vi "Initialize Kinect.vi"(8 "error in (no error)":errorcluster, 9 "Depth Image Format":T1, 10 "Color Image Format":T2, 11 "Kinect Sensor Index":i32) -> (0 "error out":errorcluster, 3 "Kinect Session out":refnum<class "Kinect Session.lvclass">)   [LabVIEW 2014, in "Kinect Library.lvlib"]
doc: "This is the basic initialization VI for the Kinect API. You may use it to connect to any Kinect sensors attached to this computer. You can provide it with the index of the Kinect which can be retrieved using the Get Device Info VI."
uses:
  Kinect Library.lvlib
  Kinect Session Class/Kinect Session.lvclass
  Kinect Type Defs/Color Image Format.ctl
  Kinect Type Defs/Depth Image Format.ctl
  Microsoft.Kinect
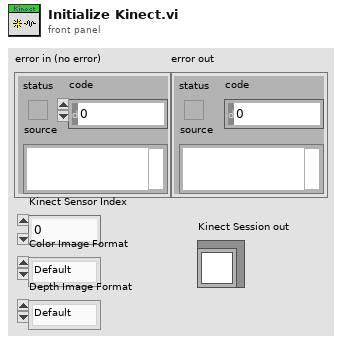
[diagram p1: front panel]
types:
  T1 = typedef "Kinect Library.lvlib/Depth Image Format.ctl" = enum16{"Default", "Undefined", "Resolution640x480Fps30", "Resolution320x240Fps30", "Resolution80x60Fps30"}
  T2 = typedef "Kinect Library.lvlib/Color Image Format.ctl" = enum16{"Default", "Undefined", "RgbResolution640x480Fps30", "RgbResolution1280x960Fps12", "YuvResolution640x480Fps15", "RawYuvResolution640x480Fps15"}
  T3 = cluster{"FramePixelDataLength":i32, "FrameWidth":i32, "FrameHeight":i32}
  T4 = cluster{"Skeleton Array":refnum<k24>[], "FrameSkeletonArrayLength":i32}
  T5 = typedef "Image Type" = u32
  T6 = typedef "IMAQ Image.ctl" = refnum<image>
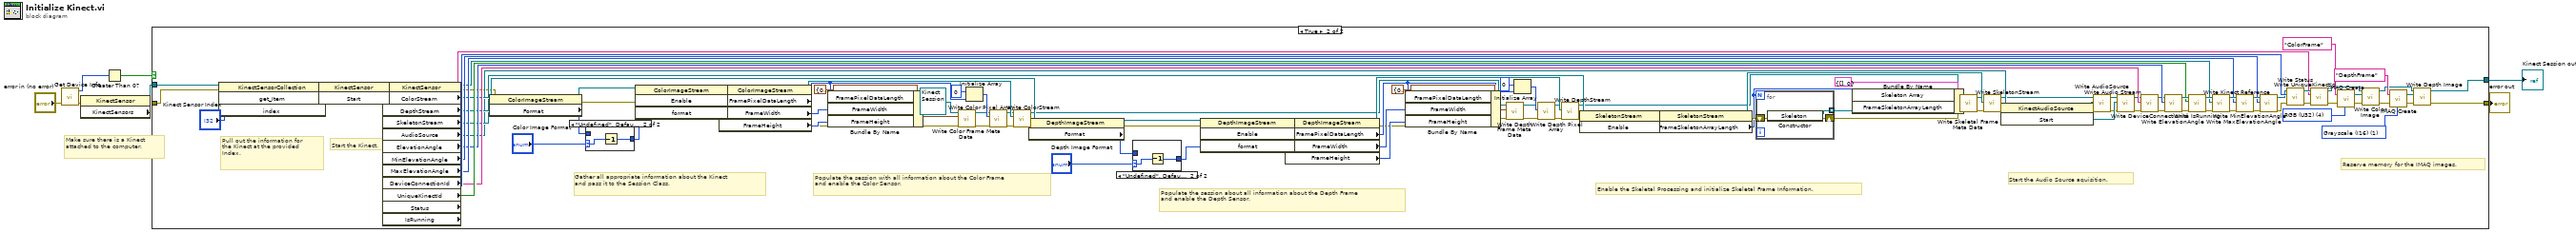
[diagram p0: block diagram]
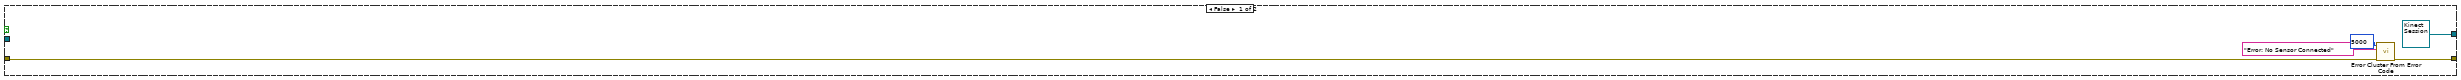
[diagram p2: hidden frame]
diagram:
  # "Make sure there is a Kinect\nattached to the computer."
  n1 = call "Get Device Info.vi"("error in (no error)"="error in (no error)") -> ("error out"=w4:errorcluster, "Number of Kinects Attached"=w8:i32)  [unwired: 8 in, 1 out]
  n2 = property class="KinectSensor"(error in=w4) -> (error out=w3:errorcluster, "KinectSensors"=w5:refnum<k24>)  [unwired: 1 in, 1 out]
  n3 = Greater Than 0?(x=w8) -> (x > 0?=w7:bool)
  n4 = case shown="True" w7 {
    tunnel: w3 -> [w11 w124]
    tunnel: w5 -> [_ w123]
    tunnel: [w10 w49] -> w1
    tunnel: [refnum<class "Kinect Session.lvclass"> refnum ("Kinect Session.lvclass") w46] -> w2
    frame False {
      n5 = call <vilib>:"Error Cluster From Error Code.vi"("error in (no error)"=w11, "error message (\"\")"="Error: No Sensor Connected" ("error message (\"\")"), "error code (0)"=5000) -> ("error out"=w10:errorcluster)  [unwired: 6 in]
    }
    frame True {
      w54 = T5 1 items=["Grayscale (U8)", "Grayscale (I16)", "Grayscale (SGL)", "Complex (CSG)", "RGB (U32)", "HSL (U32)", "RGB (U64)", "Grayscale (U16)"] ("Image Type")
      w57 = T5 4 items=["Grayscale (U8)", "Grayscale (I16)", "Grayscale (SGL)", "Complex (CSG)", "RGB (U32)", "HSL (U32)", "RGB (U64)", "Grayscale (U16)"] ("Image Type")
      # "Reserve memory for the IMAQ images."
      # "Start the Audio Source aquisition."
      # "Enable the Skeletal Processing and initialize Skeletal Frame Information."
      # "Populate the session about all information about the Depth Frame\nand enable the Depth Sensor."
      # "Populate the session with all information about the Color Frame\nand enable the Color Sensor."
      # "Gather all appropriate information about the Kinect\nand pass it to the Session Class."
      # "Start the Kinect."
      # "Pull out the information for\nthe Kinect at the provided\nIndex."
      n6 = invoke class="KinectSensorCollection" method="get_Item"(reference=w123, error in=w124, "index"="Kinect Sensor Index") -> (error out=w125:errorcluster, "get_Item"=w126:refnum<k24>)  [unwired: 1 in, 2 out]
      n7 = invoke class="KinectSensor" method="Start"(reference=w126, error in=w125) -> (reference out=w121:refnum<k24>, error out=w120:errorcluster)  [unwired: 1 in, 1 out]
      n8 = property class="KinectSensor"(reference=w121, error in=w120) -> (reference out=w110:refnum<k24>, error out=w93:errorcluster, "ColorStream"=w104:refnum<k24>, "DepthStream"=w102:refnum<k24>, "SkeletonStream"=w98:refnum<k24>, "AudioSource"=w95:refnum<k24>, "ElevationAngle"=w108:i32, "MinElevationAngle"=w112:i32, "MaxElevationAngle"=w111:i32, "DeviceConnectionId"=w107:string, "UniqueKinectId"=w114:string, "Status"=w113:i32, "IsRunning"=w109:bool)
      n9 = property class="ColorImageStream"(reference=w104, error in=w93) -> (reference out=w106:refnum<k24>, error out=w92:errorcluster, "Format"=w18:i32)
      n10 = case shown="\"Undefined\", Default" "Color Image Format" {
        selector: "Color Image Format" -> [_ w132]
        tunnel: w18 -> [w130 _]
        tunnel: [w130 w131] -> w17
        frame "Default" {
        }
        frame "Undefined", Default {
          n11 = Decrement(x=w132) -> (x-1=w131:T2)
        }
      }
      n12 = invoke class="ColorImageStream" method="Enable"(reference=w106, error in=w92, "format"=w17) -> (reference out=w105:refnum<k24>, error out=w91:errorcluster)  [unwired: 1 in, 2 out]
      n13 = property class="ColorImageStream"(reference=w105, error in=w91) -> (reference out=w103:refnum<k24>, error out=w34:errorcluster, "FramePixelDataLength"=w38:i32, "FrameWidth"=w37:i32, "FrameHeight"=w36:i32)
      n14 = Bundle By Name(cluster=T3 {"FramePixelDataLength"=0, "FrameWidth"=0, "FrameHeight"=0}, "FramePixelDataLength"=w38, "FrameWidth"=w37, "FrameHeight"=w36) -> (w35:T3)
      n15 = call-dynamic "Write Color Frame Meta Data.vi"("error in (no error)"=w34, "Color Frame Meta Data"=w35, "Kinect Session in"=refnum<class "Kinect Session.lvclass"> refnum ("Kinect Session.lvclass")) -> ("error out"=w33:errorcluster, "Kinect Session out"=w31:refnum<class "Kinect Session.lvclass">)  [unwired: 7 in]
      n16 = Initialize Array(u8 0, w38) -> (w66:u8[])
      n17 = call-dynamic "Write Color Pixel Array.vi"("error in (no error)"=w33, "Color Pixel Array"=w66, "Kinect Session in"=w31) -> ("error out"=w65:errorcluster, "Kinect Session out"=w64:refnum<class "Kinect Session.lvclass">)  [unwired: 7 in]
      n18 = call-dynamic "Write ColorStream.vi"("error in (no error)"=w65, "ColorStream"=w103, "Kinect Session in"=w64) -> ("error out"=w90:errorcluster, "Kinect Session out"=w27:refnum<class "Kinect Session.lvclass">)  [unwired: 7 in]
      n19 = property class="DepthImageStream"(reference=w102, error in=w90) -> (reference out=w101:refnum<k24>, error out=w89:errorcluster, "Format"=w16:i32)
      n20 = case shown="\"Undefined\", Default" "Depth Image Format" {
        selector: "Depth Image Format" -> [_ w129]
        tunnel: w16 -> [w127 _]
        tunnel: [w127 w128] -> w14
        frame "Default" {
        }
        frame "Undefined", Default {
          n21 = Decrement(x=w129) -> (x-1=w128:T1)
        }
      }
      n22 = invoke class="DepthImageStream" method="Enable"(reference=w101, error in=w89, "format"=w14) -> (reference out=w100:refnum<k24>, error out=w88:errorcluster)  [unwired: 1 in, 2 out]
      n23 = property class="DepthImageStream"(reference=w100, error in=w88) -> (reference out=w99:refnum<k24>, error out=w30:errorcluster, "FramePixelDataLength"=w42:i32, "FrameWidth"=w41:i32, "FrameHeight"=w40:i32)
      n24 = Bundle By Name(cluster=T3 {"FramePixelDataLength"=0, "FrameWidth"=0, "FrameHeight"=0}, "FramePixelDataLength"=w42, "FrameWidth"=w41, "FrameHeight"=w40) -> (w28:T3)
      n25 = call-dynamic "Write Depth Frame Meta Data.vi"("error in (no error)"=w30, "Depth Frame Meta Data"=w28, "Kinect Session in"=w27) -> ("error out"=w29:errorcluster, "Kinect Session out"=w26:refnum<class "Kinect Session.lvclass">)  [unwired: 7 in]
      n26 = Initialize Array(i16 0, w42) -> (w67:i16[])
      n27 = call-dynamic "Write Depth Pixel Array.vi"("error in (no error)"=w29, "Depth Pixel Array"=w67, "Kinect Session in"=w26) -> ("error out"=w63:errorcluster, "Kinect Session out"=w62:refnum<class "Kinect Session.lvclass">)  [unwired: 7 in]
      n28 = call-dynamic "Write DepthStream.vi"("error in (no error)"=w63, "DepthStream"=w99, "Kinect Session in"=w62) -> ("error out"=w87:errorcluster, "Kinect Session out"=w24:refnum<class "Kinect Session.lvclass">)  [unwired: 7 in]
      n29 = invoke class="SkeletonStream" method="Enable"(reference=w98, error in=w87) -> (reference out=w97:refnum<k24>, error out=w86:errorcluster)  [unwired: 1 in, 1 out]
      n30 = property class="SkeletonStream"(reference=w97, error in=w86) -> (reference out=w96:refnum<k24>, error out=w85:errorcluster, "FrameSkeletonArrayLength"=w20:i32)
      n31 = for {
        N: w20 -> [_]
        tunnel: [w135] -> w44 mode=indexing
        shift-right: [w133] -> w22
        shift-left: w85 -> [w134]
        n32 = constructor class="Skeleton"(error in=w134) -> (reference out=w135:refnum<k24>, error out=w133:errorcluster)  [unwired: 2 in, 1 out]
      }
      n33 = Bundle By Name(cluster=T4 {"Skeleton Array"=[], "FrameSkeletonArrayLength"=0}, "Skeleton Array"=w44, "FrameSkeletonArrayLength"=w20) -> (w25:T4)
      n34 = call-dynamic "Write Skeletal Frame Meta Data.vi"("error in (no error)"=w22, "Skeletal Frame Meta Data"=w25, "Kinect Session in"=w24) -> ("error out"=w21:errorcluster, "Kinect Session out"=w23:refnum<class "Kinect Session.lvclass">)  [unwired: 7 in]
      n35 = call-dynamic "Write SkeletonStream.vi"("error in (no error)"=w21, "SkeletonStream"=w96, "Kinect Session in"=w23) -> ("error out"=w82:errorcluster, "Kinect Session out"=w84:refnum<class "Kinect Session.lvclass">)  [unwired: 7 in]
      n36 = invoke class="KinectAudioSource" method="Start"(reference=w95, error in=w82) -> (reference out=w94:refnum<k24>, error out=w71:errorcluster, "Start"=w72:refnum<k24>)  [unwired: 1 in]
      n37 = call-dynamic "Write AudioSource.vi"("error in (no error)"=w71, "AudioSource"=w94, "Kinect Session in"=w84) -> ("error out"=w70:errorcluster, "Kinect Session out"=w68:refnum<class "Kinect Session.lvclass">)  [unwired: 7 in]
      n38 = call-dynamic "Write Audio Stream.vi"("error in (no error)"=w70, "Audio Stream"=w72, "Kinect Session in"=w68) -> ("error out"=w69:errorcluster, "Kinect Session out"=w61:refnum<class "Kinect Session.lvclass">)  [unwired: 7 in]
      n39 = call-dynamic "Write DeviceConnectionId.vi"("error in (no error)"=w69, "DeviceConnectionId"=w107, "Kinect Session in"=w61) -> ("error out"=w81:errorcluster, "Kinect Session out"=w60:refnum<class "Kinect Session.lvclass">)  [unwired: 7 in]
      n40 = call-dynamic "Write ElevationAngle.vi"("error in (no error)"=w81, "ElevationAngle"=w108, "Kinect Session in"=w60) -> ("error out"=w80:errorcluster, "Kinect Session out"=w119:refnum<class "Kinect Session.lvclass">)  [unwired: 7 in]
      n41 = call-dynamic "Write IsRunning.vi"("error in (no error)"=w80, "IsRunning"=w109, "Kinect Session in"=w119) -> ("error out"=w79:errorcluster, "Kinect Session out"=w118:refnum<class "Kinect Session.lvclass">)  [unwired: 7 in]
      n42 = call-dynamic "Write Kinect Reference.vi"("error in (no error)"=w79, "Kinect Reference"=w110, "Kinect Session in"=w118) -> ("error out"=w78:errorcluster, "Kinect Session out"=w117:refnum<class "Kinect Session.lvclass">)  [unwired: 7 in]
      n43 = call-dynamic "Write MaxElevationAngle.vi"("error in (no error)"=w78, "MaxElevationAngle"=w111, "Kinect Session in"=w117) -> ("error out"=w77:errorcluster, "Kinect Session out"=w116:refnum<class "Kinect Session.lvclass">)  [unwired: 7 in]
      n44 = call-dynamic "Write MinElevationAngle.vi"("error in (no error)"=w77, "MinElevationAngle"=w112, "Kinect Session in"=w116) -> ("error out"=w76:errorcluster, "Kinect Session out"=w83:refnum<class "Kinect Session.lvclass">)  [unwired: 7 in]
      n45 = call-dynamic "Write Status.vi"("error in (no error)"=w76, "Status"=w113, "Kinect Session in"=w83) -> ("error out"=w75:errorcluster, "Kinect Session out"=w115:refnum<class "Kinect Session.lvclass">)  [unwired: 7 in]
      n46 = call-dynamic "Write UniqueKinectId.vi"("error in (no error)"=w75, "UniqueKinectId"=w114, "Kinect Session in"=w115) -> ("error out"=w56:errorcluster, "Kinect Session out"=w48:refnum<class "Kinect Session.lvclass">)  [unwired: 7 in]
      n47 = call "IMAQ Create"("Image Name"="ColorFrame", "Image Type"=w57, "error in (no error)"=w56) -> ("New Image"=w59:T6, "error out"=w55:errorcluster)  [unwired: 2 in]
      n48 = call-dynamic "Write Color Image.vi"("error in (no error)"=w55, "Image"=w59, "Kinect Session in"=w48) -> ("error out"=w51:errorcluster, "Kinect Session out"=w47:refnum<class "Kinect Session.lvclass">)  [unwired: 7 in]
      n49 = call "IMAQ Create"("Image Name"="DepthFrame", "Image Type"=w54, "error in (no error)"=w51) -> ("New Image"=w52:T6, "error out"=w50:errorcluster)  [unwired: 2 in]
      n50 = call-dynamic "Write Depth Image.vi"("error in (no error)"=w50, "Image"=w52, "Kinect Session in"=w47) -> ("error out"=w49:errorcluster, "Kinect Session out"=w46:refnum<class "Kinect Session.lvclass">)  [unwired: 7 in]
    }
  }
  "Kinect Session out" <- w2
  "error out" <- w1
